vi "SaveVIArray.vi"(6 "Total Iteration Progress":dbl, 7 "Project":refnum<vi>, 8 "error in (no error)":errorcluster, 9 "Panels Minimized":string[](array[string]), 10 "Panels Open":string[](array[string]), 11 "VIs In":refnum<vi>[](array[refnum])) -> (0 "error out":errorcluster)   [LabVIEW 2016, in "NI_NPW_Project Copying.lvlib"]
uses:
  <resource>/dialog/NewProjectWizard/Project Copying/NI_NPW_Project Copying.lvlib
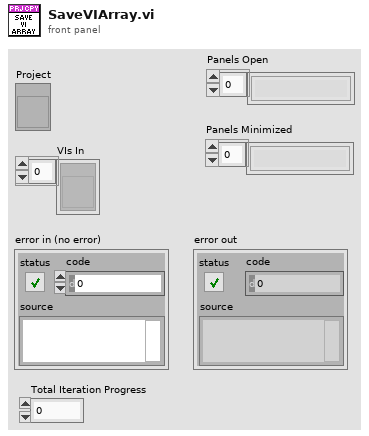
[diagram p1: front panel]
types:
  T1 = enum32{"Invalid", "Standard", "Closed", "Hidden", "Minimized", "Maximized"}
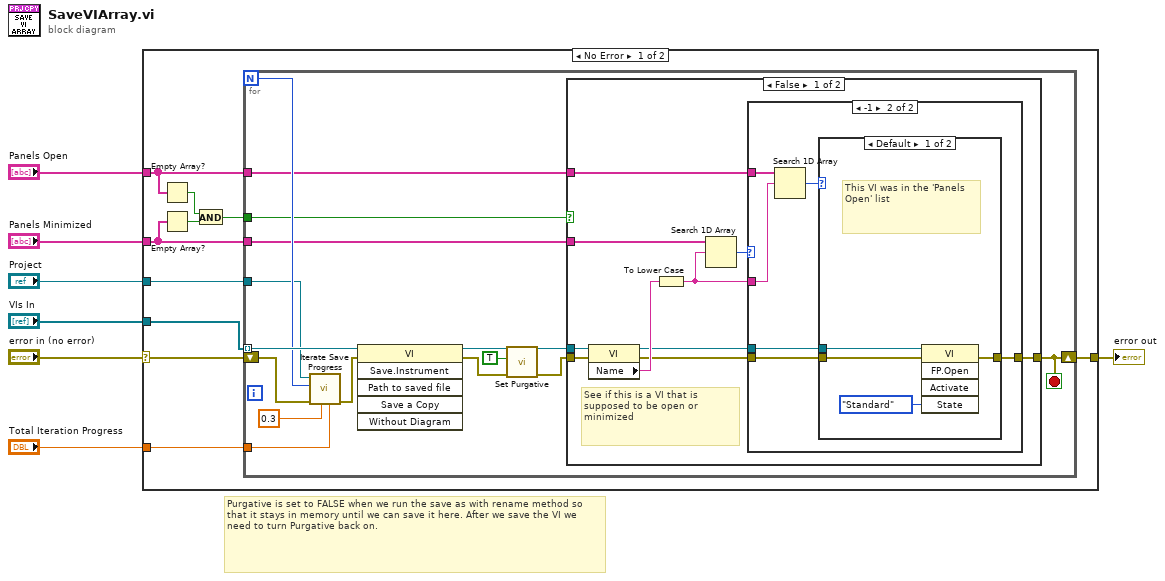
[diagram p0: block diagram]
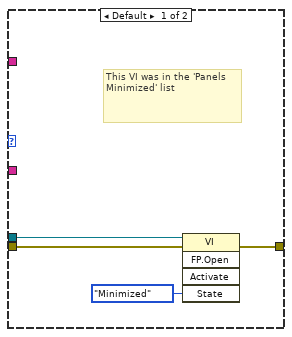
[diagram p2: hidden frame]
diagram:
  # "Purgative is set to FALSE when we run the save as with rename method so that it stays in memory until we can save it here. After we save the VI we need to turn Purgative back on."
  n1 = case shown="No Error" "error in (no error)" {
    selector: "error in (no error)" -> [w15 w60]
    tunnel: "VIs In" -> [w17 _]
    tunnel: [w16 w60] -> w6
    tunnel: "Total Iteration Progress" -> [w14 _]
    tunnel: "Project" -> [w13 _]
    tunnel: "Panels Open" -> [w12 _]
    tunnel: "Panels Minimized" -> [w11 _]
    frame No Error {
      n2 = Empty Array?(array=w12) -> (empty?=w10:bool)
      n3 = Empty Array?(array=w11) -> (empty?=w9:bool)
      n4 = And(x=w10, y=w9) -> (x .and. y?=w8:bool)
      n5 = for {
        N -> [w29]
        tunnel: w17 -> [w33] mode=indexing
        shift-right: [w19] -> w16
        shift-left: w15 -> [w32]
        tunnel: w14 -> [w28]
        tunnel: w13 -> [w27]
        tunnel: w12 -> [w24]
        tunnel: w11 -> [w23]
        tunnel: w8 -> [w22]
        stop <- w19 stop-if-true
        n6 = call <resource>:"Iterate Save Progress.vi"("Total Iteration Progress"=w28, "This Task's Percentage"=0.3, "error in (no error)"=w32, "Total Iterations (this task)"=w29, "Project"=w27) -> ("error out"=w31:errorcluster)  [unwired: 6 in]
        n7 = invoke class="VI" method="Save.Instrument"(reference=w33, error in=w31) -> (reference out=w26:refnum<vi>, error out=w25:errorcluster)  [unwired: 4 in, 4 out]
        n8 = call <resource>:"Set Purgative.vi"("error in (no error)"=w25, "Purgative?"=TRUE, "VI in"=w26) -> ("error out"=w21:errorcluster, "VI out"=w20:refnum<vi>)  [unwired: 7 in]
        n9 = case shown="False" w22 {
          tunnel: w24 -> [w38 _]
          tunnel: w23 -> [w40 _]
          tunnel: w21 -> [w42 w59]
          tunnel: w20 -> [w43 _]
          tunnel: [w35 w59] -> w19
          frame False {
            # "See if this is a VI that is supposed to be open or minimized"
            n10 = property class="VI"(reference=w43, error in=w42) -> (reference out=w36:refnum<vi>, error out=w37:errorcluster, "Name"=w41:string)
            n11 = To Lower Case(string=w41) -> (all lower case string=w34:string)
            n12 = Search 1D Array(1D array=w40, element=w34) -> (index of element=w39:i32)  [unwired: 1 in]
            n13 = case shown="-1" w39 {
              tunnel: w38 -> [_ w50]
              tunnel: w37 -> [w46 w52]
              tunnel: w36 -> [w47 w53]
              tunnel: [w44 w51] -> w35
              tunnel: w34 -> [_ w49]
              frame Default {
                # "This VI was in the 'Panels Minimized' list"
                n14 = invoke class="VI" method="FP.Open"(reference=w47, error in=w46, "State"=T1."Minimized") -> (error out=w44:errorcluster)  [unwired: 2 in, 4 out]
              }
              frame -1 {
                n15 = Search 1D Array(1D array=w50, element=w49) -> (index of element=w48:i32)  [unwired: 1 in]
                n16 = case shown="Default" w48 {
                  tunnel: w53 -> [w57 _]
                  tunnel: w52 -> [w56 w58]
                  tunnel: [w54 w58] -> w51
                  frame Default {
                    # "This VI was in the 'Panels Open' list"
                    n17 = invoke class="VI" method="FP.Open"(reference=w57, error in=w56, "State"=T1."Standard") -> (error out=w54:errorcluster)  [unwired: 2 in, 4 out]
                  }
                  frame -1 {
                    # "This VI was in neither list"
                  }
                }
              }
            }
          }
          frame True {
            # "No meta data for leaving any panels open or minimized"
          }
        }
      }
    }
    frame Error {
    }
  }
  "error out" <- w6
